vi "Reset_HP3457.vi"(8 "error in":errorcluster) -> (0 "error out":errorcluster)   [LabVIEW 2020]
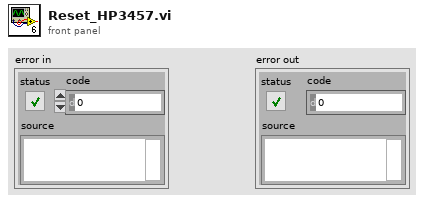
[diagram p1: front panel]
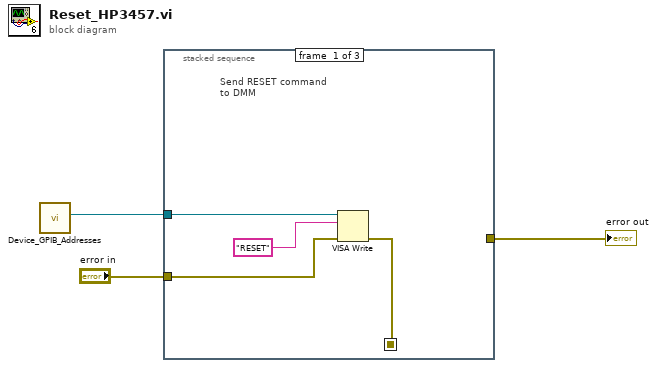
[diagram p0: block diagram]
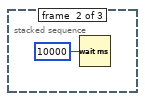
[diagram p2: hidden frame]
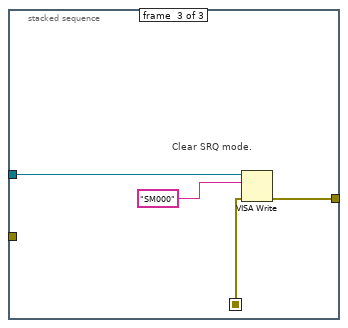
[diagram p3: hidden frame]
diagram:
  n1 = call "Device_GPIB_Addresses.vi"() -> ("HP 3457A Address"=w1:refnum<visa-resource-name>)  [unwired: 9 in, 2 out]
  n2 = stacked-sequence {
    seq-local: [w4 _ _] -> [_ _ w9]
    tunnel: [_ _ w10] -> w3
    tunnel: "error in" -> [w5 _ _]
    tunnel: w1 -> [w7 _ w11]
    frame #0 {
      # "Send RESET command\nto DMM"
      n3 = VISA Write(VISA resource name=w7, write buffer="RESET" ("data"), error in (no error)=w5) -> (error out=w4:errorcluster)  [unwired: 2 out]
    }
    frame #1 {
      n4 = Wait (ms)(milliseconds to wait=u32 10000) -> ()  [unwired: 1 out]
    }
    frame #2 {
      # "Clear SRQ mode."
      n5 = VISA Write(VISA resource name=w11, write buffer="SM000", error in (no error)=w9) -> (error out=w10:errorcluster)  [unwired: 2 out]
    }
  }
  "error out" <- w3
